vi "GetRrogInfo.vi"(8 "error in (no error)":errorcluster, 11 "RampProgramModel in":refnum<class "RampProgramModel.lvclass">) -> (0 "error out":errorcluster, 1 "Cooling rate (°C/min)":dbl, 2 "SP (°C)":dbl, 3 "RampProgramModel out":refnum<class "RampProgramModel.lvclass">, 4 "Dwell Time @ SP (sec)":u32)   [LabVIEW 2015, in "RampProgramModel.lvclass"]
uses:
  RampProgramModel.lvclass
  RampProgramModel.lvclass/RampProgramModel.ctl
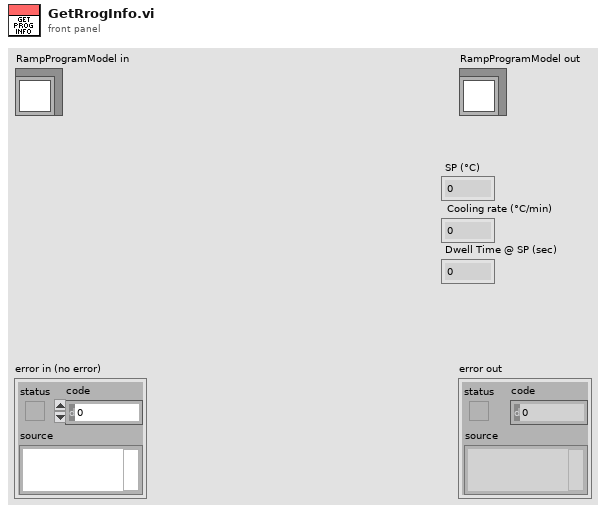
[diagram p1: front panel]
types:
  T1 = cluster{"SP (°C)":dbl, "Cooling rate (°C/min)":dbl, "Dwell Time @ SP (sec)":u32}[]
  T2 = cluster{"SP (°C)":dbl, "Cooling rate (°C/min)":dbl, "Dwell Time @ SP (sec)":u32}
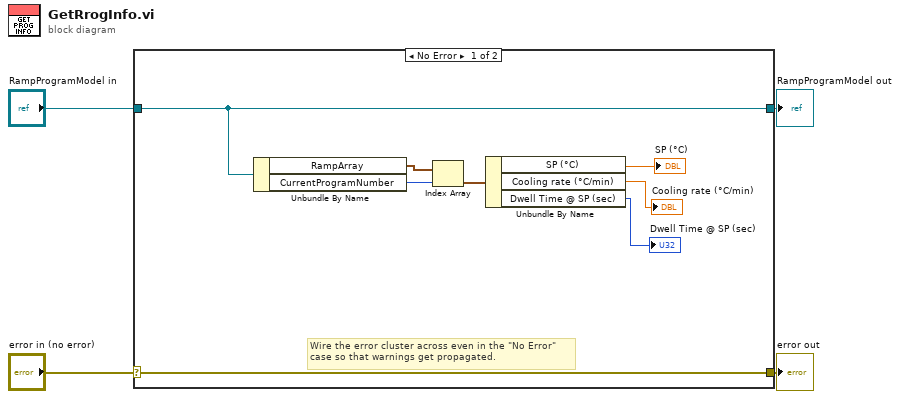
[diagram p0: block diagram]
diagram:
  n1 = case shown="No Error" "error in (no error)" {
    selector: "error in (no error)" -> [w12 w14]
    tunnel: [w12 w14] -> w3
    tunnel: [w11 w13] -> w1
    tunnel: "RampProgramModel in" -> [w11 w13]
    frame No Error {
      # "Wire the error cluster across even in the \"No Error\"\ncase so that warnings get propagated."
      n2 = Unbundle By Name(w11) -> ("RampArray"=w10:T1, "CurrentProgramNumber"=w9:u32)
      n3 = Index Array(array=w10, index=w9) -> (element=w8:T2)
      n4 = Unbundle By Name(w8) -> ("SP (°C)"=→"SP (°C)":dbl, "Cooling rate (°C/min)"=→"Cooling rate (°C/min)":dbl, "Dwell Time @ SP (sec)"=→"Dwell Time @ SP (sec)":u32)
    }
    frame Error {
    }
  }
  "error out" <- w3
  "RampProgramModel out" <- w1
